vi "ErrorConnectID.vi"(8 "ConnectArrayIN":T1(array[cluster]), 11 "ConnectIDin":refnum<k5>) -> (1 "Error":errorcluster, 2 "Address":string, 3 "ConnectIDout":refnum<k5>)   [LabVIEW 2011]
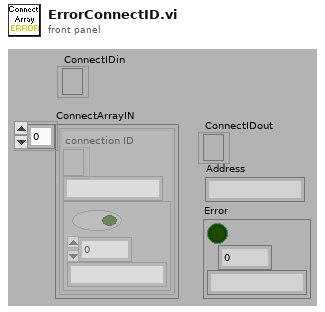
[diagram p1: front panel]
types:
  T1 = cluster{"connection ID":refnum<k5>, string, errorcluster}[]
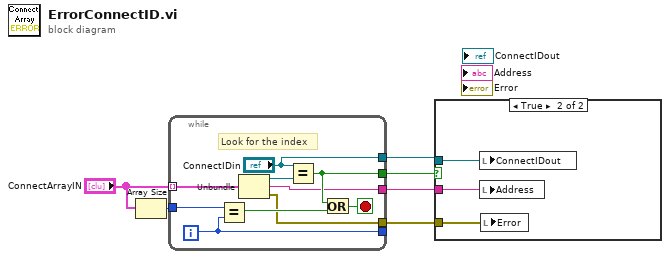
[diagram p0: block diagram]
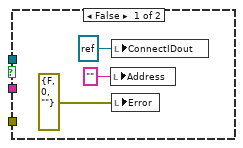
[diagram p2: hidden frame]
diagram:
  n1 = Array Size(array="ConnectArrayIN") -> (size(s)=w5:i32)
  n2 = while {
    tunnel: "ConnectArrayIN" -> [w16] mode=indexing
    tunnel: w5 -> [w13]
    tunnel: [w11] -> w3
    tunnel: [w10] -> _
    tunnel: [w9] -> w2
    tunnel: ["ConnectIDin"] -> w4
    tunnel: [w7] -> w1
    i -> [w10]
    stop <- w12 stop-if-true
    # "Look for the index"
    n3 = Equal?(x=w13, y=w10) -> (x = y?=w14:bool)
    n4 = Unbundle(w16) -> ("connection ID"=w15:refnum<k5>, w9:string, w7:errorcluster)
    n5 = Equal?(x="ConnectIDin", y=w15) -> (x = y?=w11:bool)
    n6 = Or(x=w11, y=w14) -> (x .or. y?=w12:bool)
  }
  n7 = case shown="True" w3 {
    tunnel: w4 -> [_ w22]
    tunnel: w2 -> [_ w21]
    tunnel: w1 -> [_ w20]
    frame False {
      n8 = local write "Address"("" ("Address")) -> ()
      n9 = local write "ConnectIDout"(refnum<k5> refnum ("ConnectIDout")) -> ()
      n10 = local write "Error"(errorcluster {FALSE, 0, ""} ("Error")) -> ()
    }
    frame True {
      n11 = local write "ConnectIDout"(w22) -> ()
      n12 = local write "Address"(w21) -> ()
      n13 = local write "Error"(w20) -> ()
    }
  }
